vi "Get Setpoint.vi"(8 "error in (no error)":errorcluster, 11 "Eurotherm 3200 PID Controller in":refnum<class "Eurotherm 3200 PID Controller.lvclass">) -> (0 "error out":errorcluster, 3 "Eurotherm 3200 PID Controller out":refnum<class "Eurotherm 3200 PID Controller.lvclass">)   [LabVIEW 2011, in "Eurotherm 3200 PID Controller.lvclass"]
uses:
  Eurotherm 3200 PID Controller.lvclass
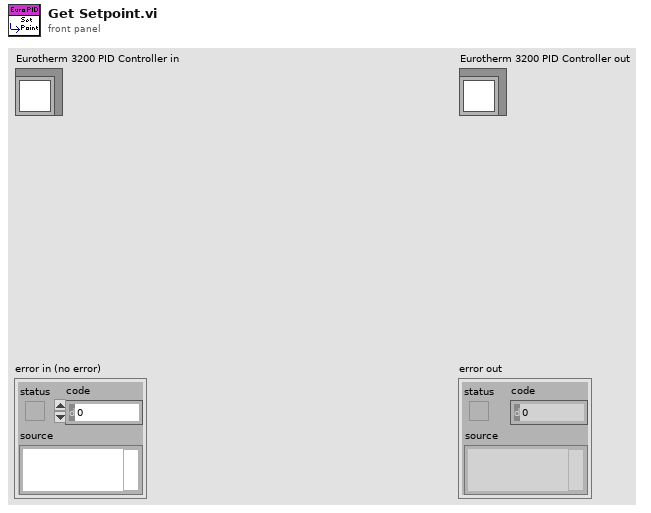
[diagram p1: front panel]
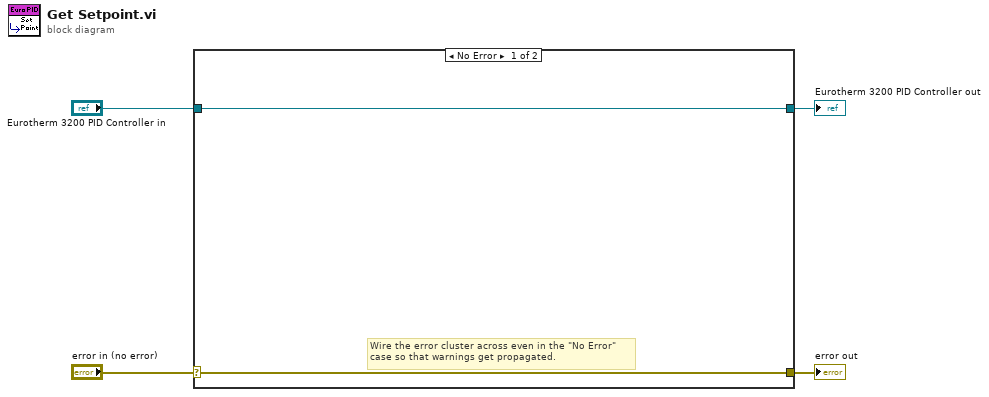
[diagram p0: block diagram]
diagram:
  n1 = case shown="No Error" "error in (no error)" {
    selector: "error in (no error)" -> [w5 w8]
    tunnel: [w5 w8] -> w3
    tunnel: [w6 w7] -> w1
    tunnel: "Eurotherm 3200 PID Controller in" -> [w6 w7]
    frame No Error {
      # "Wire the error cluster across even in the \"No Error\"\ncase so that warnings get propagated."
    }
    frame Error {
    }
  }
  "error out" <- w3
  "Eurotherm 3200 PID Controller out" <- w1
